vi "Min Max Slider Facade.vi"(0 "Data In":T5, 2 "Display State In":T3, 3 "Container State":T4) -> (6 "Data Out":T5, 7 "Display State Out":T3, 8 "Action":T2)   [LabVIEW 2012, in "Min Max Slider XControl.xctl"]
uses:
  Min Max Slider XControl.xctl
  Min Max Slider Data.ctl
  <vilib>/_xctls/Container State.ctl
  Min Max Slider State.ctl
  <vilib>/_xctls/Action.ctl
  <vilib>/_xctls/XControlSupport.lvlib
panel:
  in  "Current State":T1(ring)
  in  "Max Button":bool
  in  "Min Button":bool
  in  "Slide":dbl(slide) scale=0.0..10.0
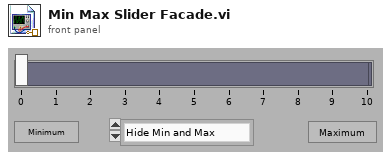
[diagram p1: front panel]
types:
  T1 = enum16{"Hide Min and Max", "Show Min", "Show Max", "Show Min and Max"}
  T2 = typedef "XControlSupport.lvlib/Action.ctl" = cluster{"Data Changed?":bool, "State Changed?":bool, "Action Name":string}
  T3 = typedef "Min Max Slider XControl.xctl/Min Max Slider State.ctl" = cluster{"Current State":enum16{"Hide Min and Max", "Show Min", "Show Max", "Show Min and Max"}}
  T4 = typedef "XControlSupport.lvlib/Container State.ctl" = cluster{"Indicator?":bool, "Run Mode?":bool, " Refnum":refnum<vi>}
  T5 = typedef "Min Max Slider XControl.xctl/Min Max Slider Data.ctl" = dbl
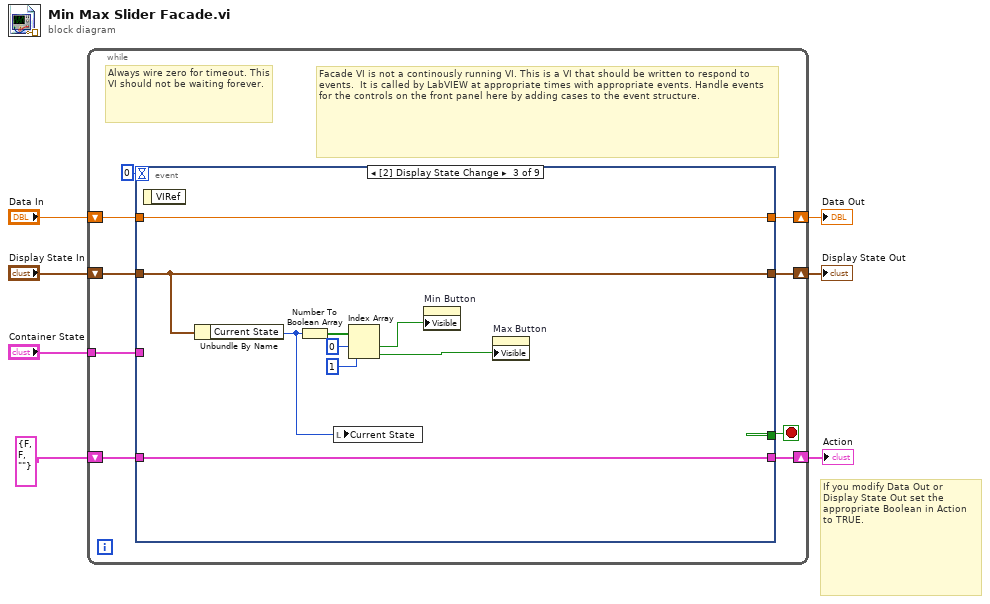
[diagram p0: block diagram]
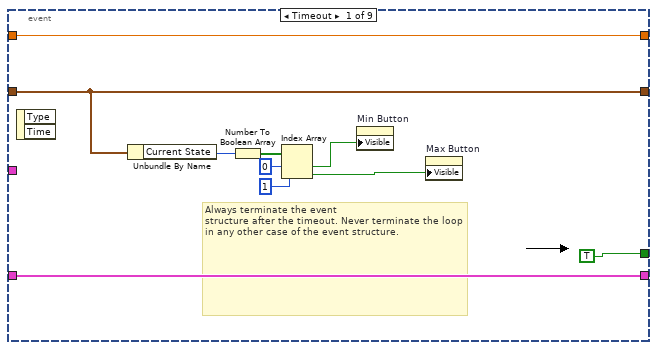
[diagram p2: hidden frame]
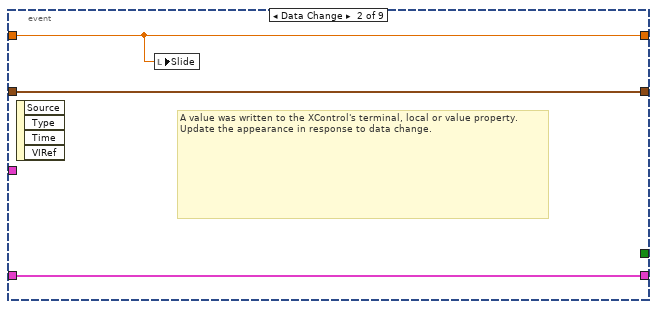
[diagram p3: hidden frame]
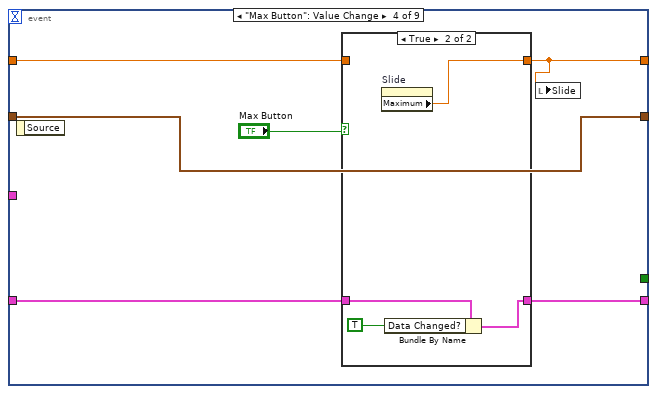
[diagram p4: hidden frame]
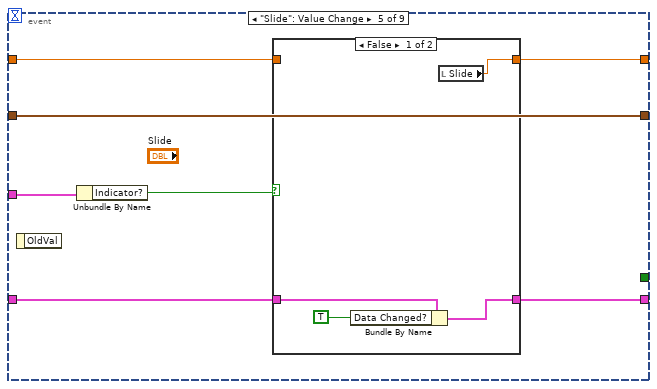
[diagram p6: hidden frame]
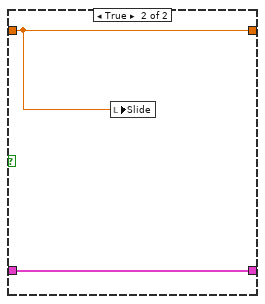
[diagram p7: hidden frame]
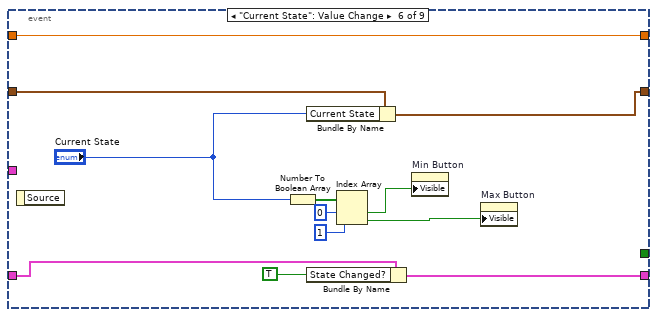
[diagram p8: hidden frame]
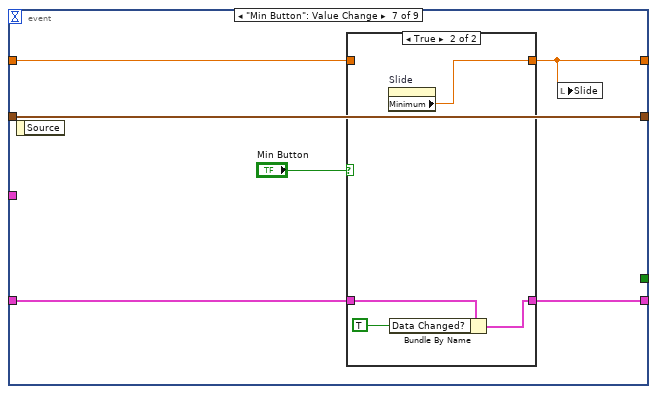
[diagram p9: hidden frame]
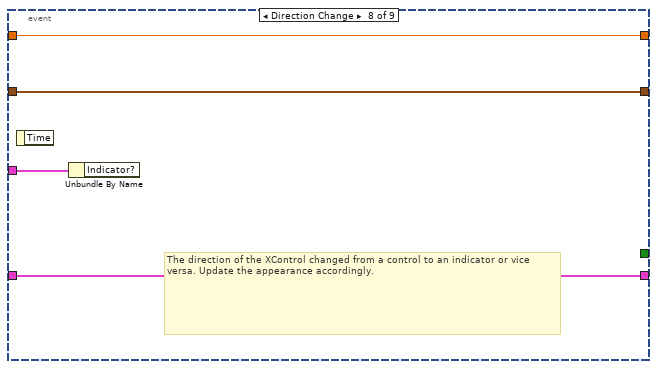
[diagram p11: hidden frame]
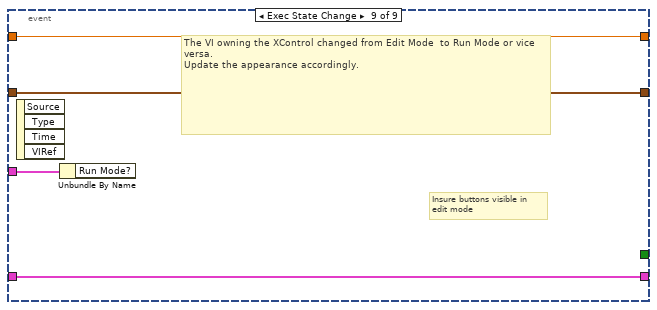
[diagram p12: hidden frame]
diagram:
  # "If you modify Data Out or\nDisplay State Out set the\nappropriate Boolean in Action\nto TRUE."
  n1 = while {
    shift-right: [w15] -> w4
    shift-left: "Display State In" -> [w16]
    tunnel: "Container State" -> [w12]
    shift-right: [w10] -> w7
    shift-left: "Data In" -> [w11]
    shift-right: [w8] -> w2
    shift-left: T2 {"Data Changed?"=FALSE, "State Changed?"=FALSE, "Action Name"=""} ("Action") -> [w9]
    stop <- w14 stop-if-true
    # "Facade VI is not a continously running VI. This is a VI that should be written to respond to events.  It is called by LabVIEW at appropriate times with appropriate events. Handle events for the controls on the front panel here by adding cases to the event structure."
    # "Always wire zero for timeout. This\nVI should not be waiting forever."
    n2 = event shown="[2] Display State Change" {
      selector: _ -> [_ _ _ _ _ _ _ _ _]
      dyn-events: _ -> [_ _ _ _ _ _ _ _ _]
      timeout: 0 -> [_ _ _ _ _ _ _ _ _]
      tunnel: w16 -> [w17 w29 w31 w42 w55 w71 w78 w88 w94]
      tunnel: [w17 w29 w31 w42 w55 w70 w78 w88 w94] -> w15
      tunnel: [TRUE _ _ _ _ _ _ _ _] -> w14
      tunnel: w12 -> [_ _ _ _ w54 _ _ w91 w95]
      tunnel: w11 -> [w24 w27 w38 w43 w51 w72 w81 w90 w93]
      tunnel: [w24 w27 w38 w39 w52 w72 w76 w90 w93] -> w10
      tunnel: [w25 w28 w37 w40 w56 w73 w79 w89 w92] -> w8
      tunnel: w9 -> [w25 w28 w37 w41 w57 w74 w80 w89 w92]
      event Timeout {
        # "Always terminate the event\nstructure after the timeout. Never terminate the loop in any other case of the event structure."
        n3 = event-data() -> ()  [unwired: 1 in, 2 out]
        n4 = Unbundle By Name(w17) -> ("Current State"=w18:T1)
        n5 = Number To Boolean Array(number=w18) -> (Boolean array=w23:bool[])
        n6 = Index Array(array=w23, index #1=0 ("index"), index #2=1 ("index")) -> (element #1=w20:bool, element #2=w19:bool)
        n7 = property on="Min Button" class="Bool"("Visible"=w20) -> ()  [unwired: 2 in, 2 out]
        n8 = property on="Max Button" class="Bool"("Visible"=w19) -> ()  [unwired: 2 in, 2 out]
      }
      event Data Change {
        # "A value was written to the XControl's terminal, local or value property.\nUpdate the appearance in response to data change."
        n9 = event-data() -> ()  [unwired: 1 in, 4 out]
        n10 = local write "Slide"(w27) -> ()
      }
      event Display State Change {
        n11 = event-data() -> ()  [unwired: 1 in, 1 out]
        n12 = Unbundle By Name(w31) -> ("Current State"=w30:T1)
        n13 = Number To Boolean Array(number=w30) -> (Boolean array=w36:bool[])
        n14 = local write "Current State"(w30) -> ()
        n15 = Index Array(array=w36, index #1=0 ("index"), index #2=1 ("index")) -> (element #1=w33:bool, element #2=w32:bool)
        n16 = property on="Min Button" class="Bool"("Visible"=w33) -> ()  [unwired: 2 in, 2 out]
        n17 = property on="Max Button" class="Bool"("Visible"=w32) -> ()  [unwired: 2 in, 2 out]
      }
      event "Max Button": Value Change {
        n18 = event-data() -> ()  [unwired: 1 in, 1 out]
        n19 = case shown="True" "Max Button" {
          tunnel: w43 -> [w46 _]
          tunnel: [w46 w50] -> w39
          tunnel: w41 -> [w45 w49]
          tunnel: [w45 w47] -> w40
          frame False {
          }
          frame True {
            n20 = property on="Slide" class="Slide (strict)"() -> ("Maximum"=w50:dbl)  [unwired: 2 in, 2 out]
            n21 = Bundle By Name(cluster=w49, "Data Changed?"=TRUE) -> (w47:T2)
          }
        }
        n22 = local write "Slide"(w39) -> ()
      }
      event "Slide": Value Change {
        n23 = event-data() -> ()  [unwired: 1 in, 1 out]
        n24 = Unbundle By Name(w54) -> ("Indicator?"=w53:bool)
        n25 = case shown="False" w53 {
          tunnel: w57 -> [w60 w62]
          tunnel: [w59 w62] -> w56
          tunnel: [w58 w63] -> w52
          tunnel: w51 -> [_ w63]
          frame False {
            n26 = Bundle By Name(cluster=w60, "Data Changed?"=TRUE) -> (w59:T2)
            n27 = local read "Slide"() -> (w58:dbl)
          }
          frame True {
            n28 = local write "Slide"(w63) -> ()
          }
        }
      }
      event "Current State": Value Change {
        n29 = event-data() -> ()  [unwired: 1 in, 1 out]
        n30 = Number To Boolean Array(number="Current State") -> (Boolean array=w69:bool[])
        n31 = Bundle By Name(cluster=w71, "Current State"="Current State") -> (w70:T3)
        n32 = Bundle By Name(cluster=w74, "State Changed?"=TRUE) -> (w73:T2)
        n33 = Index Array(array=w69, index #1=0 ("index"), index #2=1 ("index")) -> (element #1=w66:bool, element #2=w65:bool)
        n34 = property on="Min Button" class="Bool"("Visible"=w66) -> ()  [unwired: 2 in, 2 out]
        n35 = property on="Max Button" class="Bool"("Visible"=w65) -> ()  [unwired: 2 in, 2 out]
      }
      event "Min Button": Value Change {
        n36 = event-data() -> ()  [unwired: 1 in, 1 out]
        n37 = case shown="True" "Min Button" {
          tunnel: w81 -> [w83 _]
          tunnel: [w83 w87] -> w76
          tunnel: w80 -> [w82 w86]
          tunnel: [w82 w84] -> w79
          frame False {
          }
          frame True {
            n38 = property on="Slide" class="Slide (strict)"() -> ("Minimum"=w87:dbl)  [unwired: 2 in, 2 out]
            n39 = Bundle By Name(cluster=w86, "Data Changed?"=TRUE) -> (w84:T2)
          }
        }
        n40 = local write "Slide"(w76) -> ()
      }
      event Direction Change {
        # "The direction of the XControl changed from a control to an indicator or vice versa. Update the appearance accordingly."
        n41 = event-data() -> ()  [unwired: 1 in, 1 out]
        n42 = Unbundle By Name(w91) -> ()  [unwired: 1 out]
      }
      event Exec State Change {
        # "Insure buttons visible in\nedit mode"
        # "The VI owning the XControl changed from Edit Mode  to Run Mode or vice versa.\nUpdate the appearance accordingly."
        n43 = event-data() -> ()  [unwired: 1 in, 4 out]
        n44 = Unbundle By Name(w95) -> ()  [unwired: 1 out]
      }
    }
  }
  "Display State Out" <- w4
  "Data Out" <- w7
  "Action" <- w2
